vi "mod_FSK Deviation Measurement.vi"(0 "FM demodulated waveform in":waveform(dbl)={"t0"=timestamp(0 s since 1904-01-01), "dt"=0.0, "Y"=[]}, 1 "FSK system parameters":T1={"samples per symbol (16)"=16, "symbol map"=[], "symbol phase continuity"=enum."continuous"} {"symbol map" format="%.2f"}, 2 "samples per symbol (16)":i32=16, 5 "error in (no error)":errorcluster) -> (14 "FM demodulated waveform out":waveform(dbl), 15 "RMS FSK Deviation Measurements (Hz)":dbl[](array[numeric]), 16 "FSK Symbol Points":dbl[](array[numeric]), 19 "error out":errorcluster)   [LabVIEW 2020, in "niDMT.lvlib"]
uses:
  <vilib>/addons/Modulation/niDMT.lvlib
  <vilib>/addons/Modulation/Analog/controls/Complex Data Waveform.ctl
  <vilib>/Analysis/5stat.llb/RMS (DBL).vi
  <vilib>/addons/Modulation/niAMT.lvlib
  <vilib>/Analysis/NI_AALPro.lvlib
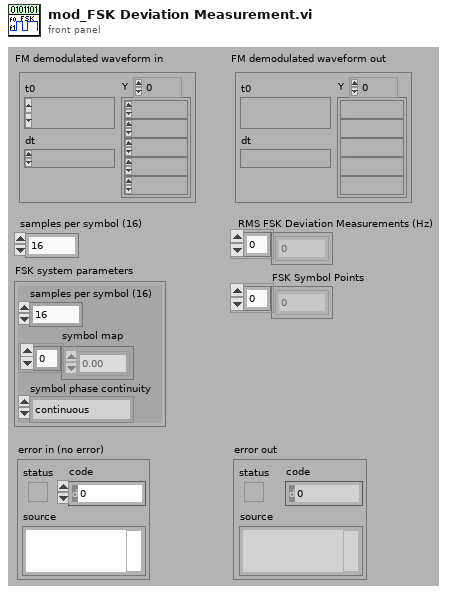
[diagram p1: front panel]
types:
  T1 = cluster{"samples per symbol (16)":i32, "symbol map":dbl[], "symbol phase continuity":enum16{"continuous", "discontinuous"}}
  T2 = typedef "niAMT.lvlib/Complex Data Waveform.ctl" = cluster{"t0":dbl, "dt":dbl, "Y":cdb[]}
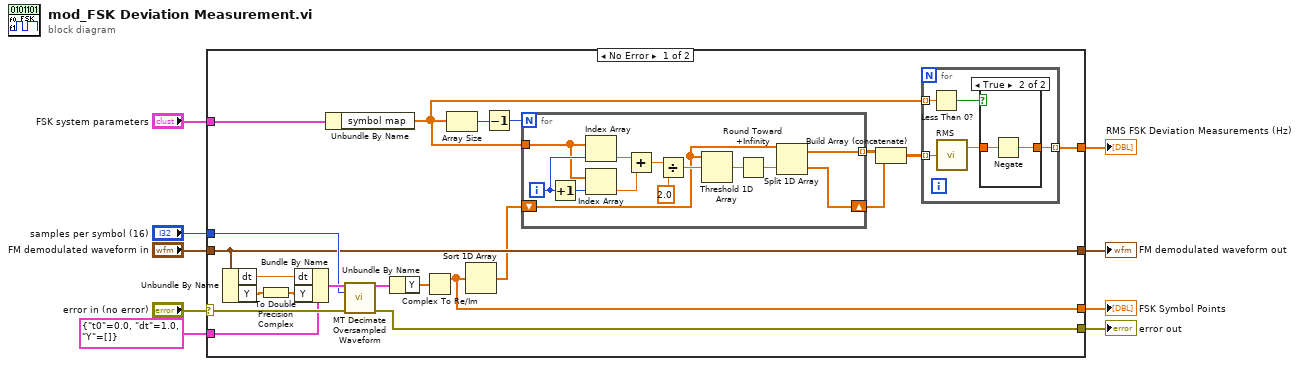
[diagram p0: block diagram]
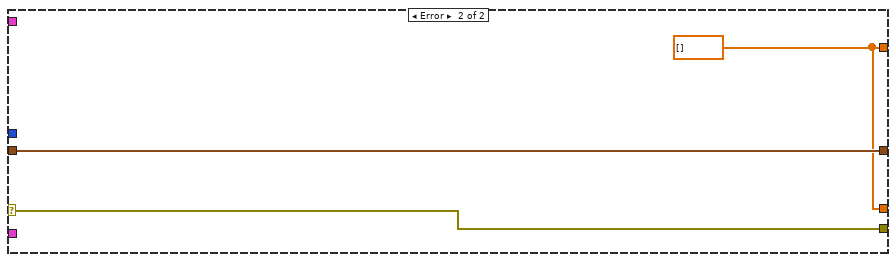
[diagram p3: hidden frame]
diagram:
  n1 = case shown="No Error" "error in (no error)" {
    selector: "error in (no error)" -> [w23 w54]
    tunnel: "FM demodulated waveform in" -> [w22 w53]
    tunnel: "samples per symbol (16)" -> [w26 _]
    tunnel: [w18 w54] -> w7
    tunnel: [w22 w53] -> w2
    tunnel: [w21 w52] -> w5
    tunnel: T2 {"t0"=0.0, "dt"=1.0, "Y"=[]} ("input complex waveform") -> [w20 _]
    tunnel: "FSK system parameters" -> [w19 _]
    tunnel: [w10 w52] -> w1
    frame No Error {
      n2 = Unbundle By Name(w22) -> ("dt"=w30:dbl, "Y"=w25:dbl[])
      n3 = To Double Precision Complex(1:w25) -> (0:w24:cdb[])
      n4 = Bundle By Name(cluster=w20, "dt"=w30, "Y"=w24) -> (w29:T2)
      n5 = Unbundle By Name(w19) -> ("symbol map"=w11:dbl[])
      n6 = call <vilib>:"MT Decimate Oversampled Waveform.vi"("input complex waveform"=w29, "decimation factor"=w26, "error in (no error)"=w23) -> ("output complex waveform"=w28:T2, "error out"=w18:errorcluster)  [unwired: 2 in, 9 out]
      n7 = Unbundle By Name(w28) -> ("Y"=w27:cdb[])
      n8 = Complex To Re/Im(x + iy=w27) -> (x=w21:dbl[])  [unwired: 1 out]
      n9 = Array Size(array=w11) -> (size(s)=w17:i32)
      n10 = Sort 1D Array(array=w21) -> (sorted array=w15:dbl[])
      n11 = Decrement(x=w17) -> (x-1=w16:i32)
      n12 = for {
        N: w16 -> [_]
        tunnel: w11 -> [w49]
        tunnel: [w41] -> w14 mode=indexing
        shift-right: [w40] -> w13
        shift-left: w15 -> [w39]
        i -> [w51]
        n13 = Increment(x=w51) -> (x+1=w50:i32)
        n14 = Index Array(array=w49, index=w51) -> (element=w47:dbl)
        n15 = Index Array(array=w49, index=w50) -> (element=w48:dbl)
        n16 = Add(x=w47, y=w48) -> (x+y=w46:dbl)
        n17 = Divide(x=w46, y=2.0) -> (x/y=w44:dbl)
        n18 = Threshold 1D Array(2:w44, 3:w39) -> (0:w43:dbl)  [unwired: 1 out]
        n19 = Round Toward +Infinity(x=w43) -> (ceil(x): smallest int >= x=w42:dbl)
        n20 = Split 1D Array(array=w39, index=w42) -> (first subarray=w41:dbl[], second subarray=w40:dbl[])
      }
      n21 = Build Array (concatenate)(w14, w13) -> (w12:dbl[][])
      n22 = for {
        tunnel: w12 -> [w35] mode=indexing
        tunnel: w11 -> [w34] mode=indexing
        tunnel: [w31] -> w10 mode=indexing
        n23 = Less Than 0?(x=w34) -> (x < 0?=w33:bool)
        n24 = call-poly <vilib>:"RMS.vi"("X"=w35) -> ("rms value"=w32:dbl)  [unwired: 1 out]
        n25 = case shown="True" w33 {
          tunnel: w32 -> [w36 w38]
          tunnel: [w36 w37] -> w31
          frame False {
          }
          frame True {
            n26 = Negate(x=w38) -> (-x=w37:dbl)
          }
        }
      }
    }
    frame Error {
      w52 = dbl[] []
    }
  }
  "error out" <- w7
  "FM demodulated waveform out" <- w2
  "FSK Symbol Points" <- w5
  "RMS FSK Deviation Measurements (Hz)" <- w1
